vi "ModbusTcp通用版.vi"(0 "IP Address":string="192.168.3.250", 1 "操作选择":string(combo), 5 "Port":u16=502, 7 "开始地址":u16, 9 "读取个数":u16, 11 "写入数组":i32[](array[numeric])=[0, 0, 0, 0, 0, 0, 0, 0, 0, 0], 12 "写继电器":bool[](array[boolean])=[FALSE, FALSE, FALSE, FALSE, FALSE, FALSE, FALSE, FALSE, FALSE], 13 "error in":errorcluster) -> (4 "读取的数据":i32[](array[numeric]), 8 "读取继电器的信号":bool[](array[boolean]), 15 "error out 2":errorcluster)   [LabVIEW 2020]
uses:
  <vilib>/NI/Modbus Library/API/Master/Modbus Master.lvclass
  C:/Program Files/National Instruments/LabVIEW 2020/vi.lib/NI/Modbus Library/API/Modbus API.lvclass
  <vilib>/NI/Modbus Library/API/Wrapper/Create TCP Master.vi
  <vilib>/NI/Modbus Library/API/Modbus API.lvclass
  <vilib>/NI/Modbus Library/API/Wrapper/API Main.lvlib
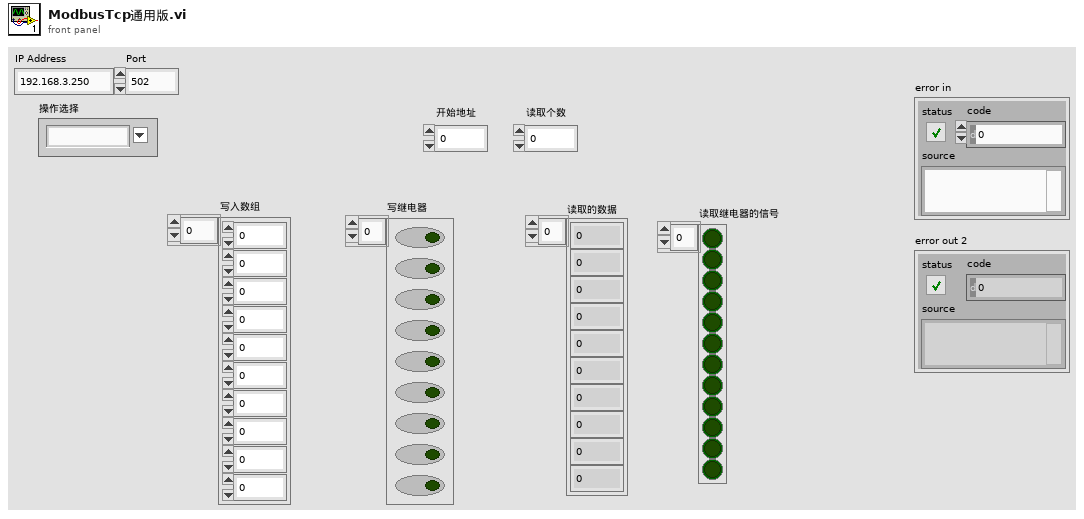
[diagram p1: front panel]
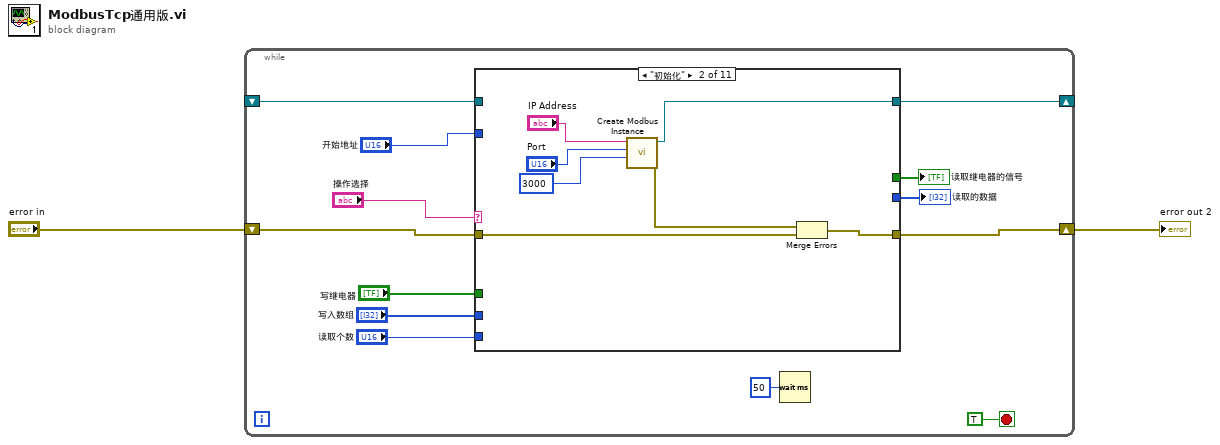
[diagram p0: block diagram]
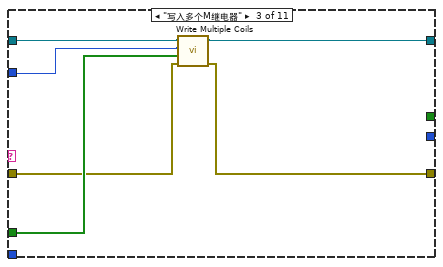
[diagram p3: hidden frame]
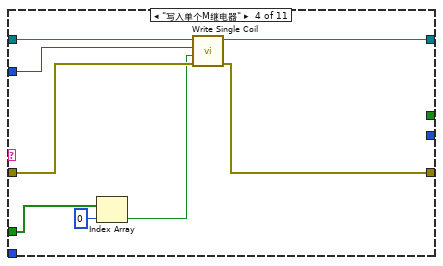
[diagram p4: hidden frame]
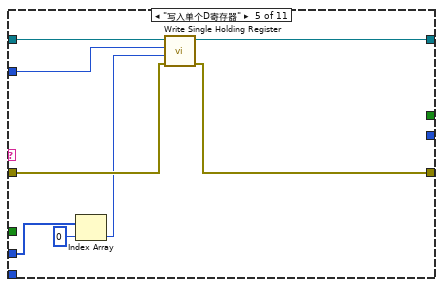
[diagram p5: hidden frame]
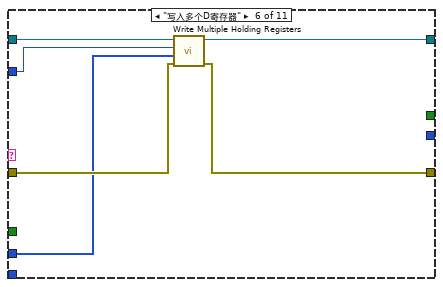
[diagram p6: hidden frame]
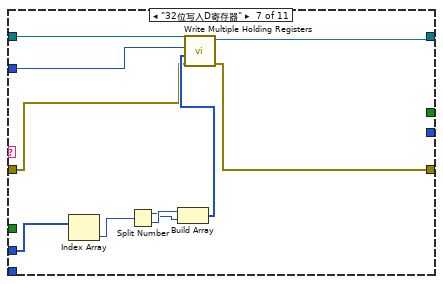
[diagram p7: hidden frame]
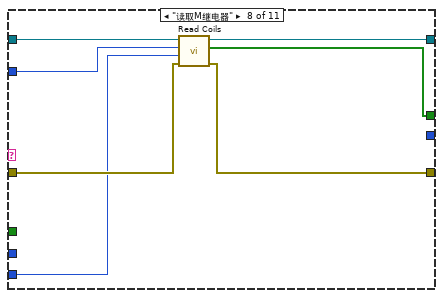
[diagram p8: hidden frame]
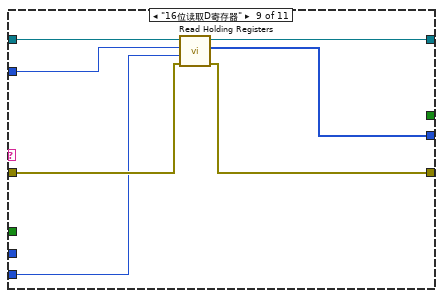
[diagram p9: hidden frame]
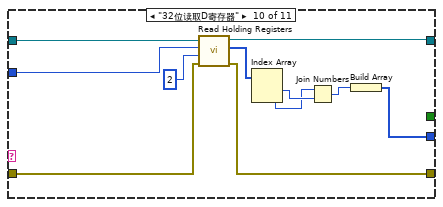
[diagram p10: hidden frame]
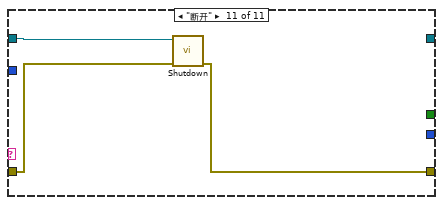
[diagram p11: hidden frame]
diagram:
  n1 = while {
    shift-right: [w13] -> w1
    shift-left: "error in" -> [w12]
    shift-right: [w5] -> _
    shift-left: _ -> [w4]
    stop <- TRUE stop-if-true
    n2 = case shown="\"初始化\"" "操作选择" {
      tunnel: [w17 w19 w25 w33 w41 w49 w53 w66 w73 w80 w88] -> w13
      tunnel: w12 -> [w17 w20 w26 w34 w42 w50 w54 w67 w74 w81 w89]
      tunnel: "开始地址" -> [_ _ w28 w31 w40 w48 w56 w65 w72 w78 _]
      tunnel: "写继电器" -> [_ _ w27 w38 _ _ _ _ _ _ _]
      tunnel: "写入数组" -> [_ _ _ _ w46 w47 w62 _ _ _ _]
      tunnel: "读取个数" -> [_ _ _ _ _ _ _ w64 w71 _ _]
      tunnel: [_ _ _ _ _ _ _ _ w70 w87 _] -> w8
      tunnel: [w16 w21 w30 w35 w43 w51 w57 w68 w75 w82 _] -> w5
      tunnel: w4 -> [w16 _ w29 w36 w44 w52 w58 w69 w76 w83 w90]
      tunnel: [_ _ _ _ _ _ _ w63 _ _ _] -> w3
      frame "默认", Default {
      }
      frame "初始化" {
        n3 = call-poly <vilib>:"Create Modbus Instance.vi"("connect timeout ms"=3000, "port (502)"="Port", "address"="IP Address") -> ("error out"=w18:errorcluster, "TCP master instance"=w21:refnum<class "Modbus Master.lvclass">)  [unwired: 7 in]
        n4 = Merge Errors(w18, w20) -> (w19:errorcluster)
      }
      frame "写入多个M继电器" {
        n5 = call-dynamic "Write Multiple Coils.vi"("error in"=w26, "coils to write"=w27, "starting address"=w28, "Modbus instance in"=w29) -> ("error out"=w25:errorcluster, "Modbus instance out"=w30:refnum<class "Modbus API.lvclass">)  [unwired: 6 in]
      }
      frame "写入单个M继电器" {
        n6 = Index Array(array=w38, index=0) -> (element=w32:bool)
        n7 = call-dynamic "Write Single Coil.vi"("error in"=w34, "coil to write"=w32, "address"=w31, "Modbus instance in"=w36) -> ("error out"=w33:errorcluster, "Modbus instance out"=w35:refnum<class "Modbus API.lvclass">)  [unwired: 6 in]
      }
      frame "写入单个D寄存器" {
        n8 = Index Array(array=w46, index=0) -> (element=w39:i32)
        n9 = call-dynamic "Write Single Holding Register.vi"("error in"=w42, "register to write"=w39, "address"=w40, "Modbus instance in"=w44) -> ("error out"=w41:errorcluster, "Modbus instance out"=w43:refnum<class "Modbus API.lvclass">)  [unwired: 6 in]
      }
      frame "写入多个D寄存器" {
        n10 = call-dynamic "Write Multiple Holding Registers.vi"("error in"=w50, "registers to write"=w47, "starting address"=w48, "Modbus instance in"=w52) -> ("error out"=w49:errorcluster, "Modbus instance out"=w51:refnum<class "Modbus API.lvclass">)  [unwired: 6 in]
      }
      frame "32位写入D寄存器" {
        n11 = Index Array(array=w62) -> (element=w61:i32)  [unwired: 1 in]
        n12 = Split Number(x=w61) -> (hi(x)=w59:u16, lo(x)=w60:u16)
        n13 = Build Array(w60, w59) -> (w55:u16[])
        n14 = call-dynamic "Write Multiple Holding Registers.vi"("error in"=w54, "registers to write"=w55, "starting address"=w56, "Modbus instance in"=w58) -> ("error out"=w53:errorcluster, "Modbus instance out"=w57:refnum<class "Modbus API.lvclass">)  [unwired: 6 in]
      }
      frame "读取M继电器" {
        n15 = call-dynamic "Read Coils.vi"("error in"=w67, "number of inputs"=w64, "starting address"=w65, "Modbus instance in"=w69) -> ("error out"=w66:errorcluster, "coils"=w63:bool[], "Modbus instance out"=w68:refnum<class "Modbus API.lvclass">)  [unwired: 5 in]
      }
      frame "16位读取D寄存器" {
        n16 = call-dynamic "Read Holding Registers.vi"("error in"=w74, "number of inputs"=w71, "starting address"=w72, "Modbus instance in"=w76) -> ("error out"=w73:errorcluster, "register values"=w70:u16[], "Modbus instance out"=w75:refnum<class "Modbus API.lvclass">)  [unwired: 5 in]
      }
      frame "32位读取D寄存器" {
        n17 = call-dynamic "Read Holding Registers.vi"("error in"=w81, "number of inputs"=u16 2 ("quantity"), "starting address"=w78, "Modbus instance in"=w83) -> ("error out"=w80:errorcluster, "register values"=w77:u16[], "Modbus instance out"=w82:refnum<class "Modbus API.lvclass">)  [unwired: 5 in]
        n18 = Index Array(array=w77) -> (element #1=w86:u16, element #2=w85:u16)  [unwired: 2 in]
        n19 = Join Numbers(hi=w85, lo=w86) -> ((hi.lo)=w84:u32)
        n20 = Build Array(w84) -> (w87:u32[])
      }
      frame "断开" {
        n21 = call-dynamic "Shutdown.vi"("error in"=w89, "Modbus instance in"=w90) -> ("error out"=w88:errorcluster)  [unwired: 9 in]
      }
    }
    "读取继电器的信号" <- w3
    "读取的数据" <- w8
    n22 = Wait (ms)(milliseconds to wait=u32 50) -> ()  [unwired: 1 out]
  }
  "error out 2" <- w1
